vi "Template_Custom Error.vi"(8 "error in":errorcluster) -> (0 "error out":errorcluster)   [LabVIEW 2020]
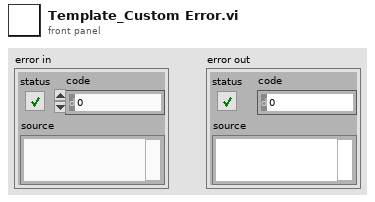
[diagram p1: front panel]
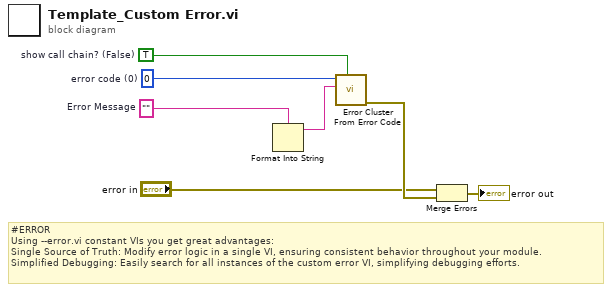
[diagram p0: block diagram]
diagram:
  w3 = 0  # error code (0)
  w1 = ""  # Error Message
  w4 = TRUE  # show call chain? (False)
  # "#ERROR\nUsing --error.vi constant VIs you get great advantages:\nSingle Source of Truth: Modify error logic in a single VI, ensuring consistent behavior throughout your module.\nSimplified Debugging: Easily search for all instances of the custom error VI, simplifying debugging efforts."
  n1 = Format Into String(format string=w1) -> (resulting string=w2:string)  [unwired: 3 in, 1 out]
  n2 = call <vilib>:"Error Cluster From Error Code.vi"("show call chain? (False)"=w4, "error message (\"\")"=w2, "error code (0)"=w3) -> ("error out"=w7:errorcluster)  [unwired: 6 in]
  n3 = Merge Errors("error in", w7) -> (→"error out":errorcluster)
